vi "Set VI Allow Debugging Property.vi"() -> ()   [LabVIEW 2016]
doc: "A wrapper engine for setting separate compiled code for all VIs in a folder."
uses:
  <vilib>/Utility/error.llb/DialogType.ctl
  SLL Queued State Machine/Queue Driver/Create Queue.vi
  SLL Queued State Machine/Queue Driver/Enqueue an Item to Queue.vi
  SLL Queued State Machine/Queue Driver/Dequeue Queue.vi
  SLL Queued State Machine/Queue Driver/Enqueue N Items.vi
  SLL Queued State Machine/Queue Driver/Flush Queue.vi
  SLL Queued State Machine/Queue Driver/Release Queue.vi
  SLL Queued State Machine/SLL QSM.lvlib
panel:
  out "Progress":i32(slide) scale=0.0..10.0
  in  "Allow Debugging?":bool
  in  "Folder Path":path
  out "Status":string
  in  "Run":bool
  # "Set VI Allow Debugging Property"
  # "Sets the allow debugging property for the VIs in the folder"
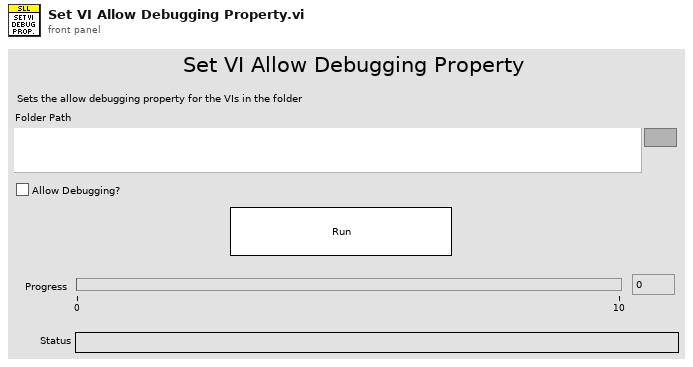
[diagram p1: front panel]
types:
  T1 = typedef "DialogType.ctl" = u16
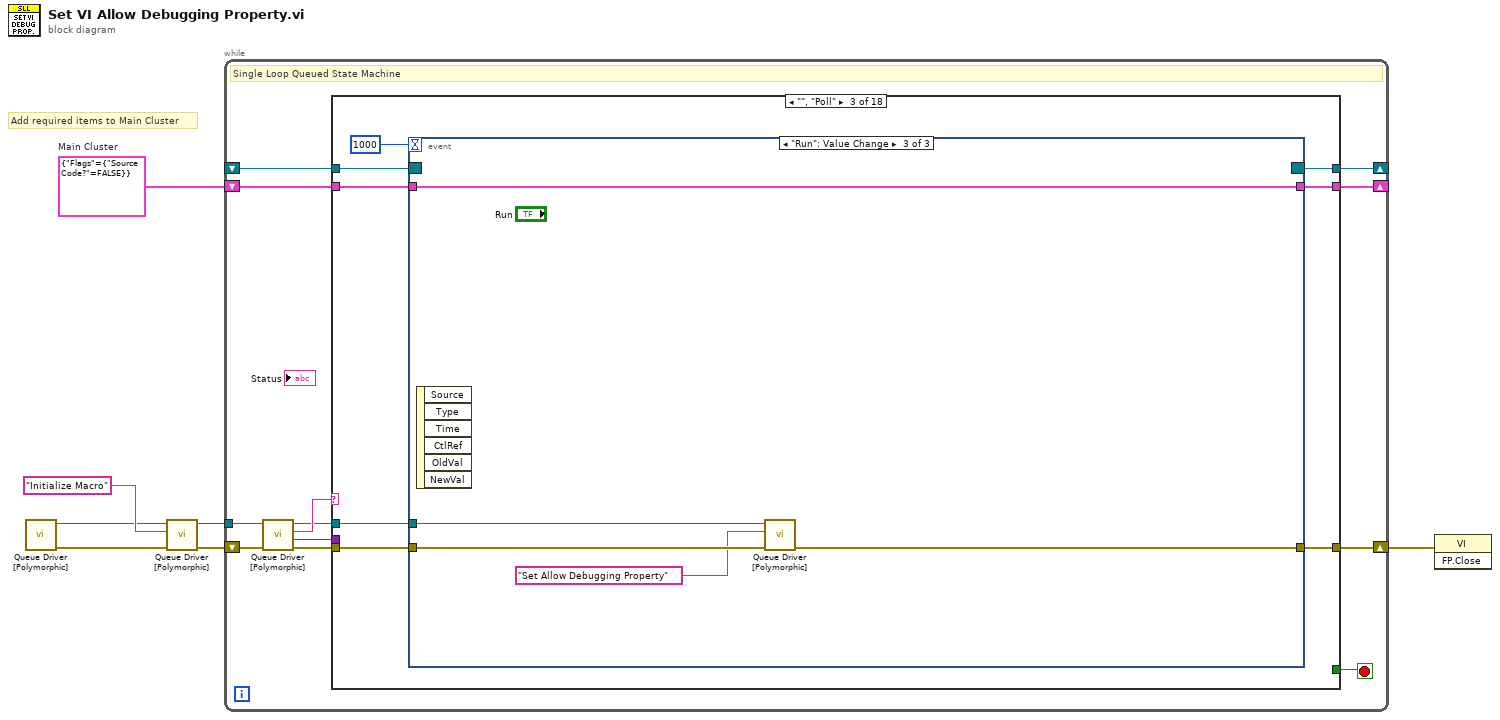
[diagram p0: block diagram]
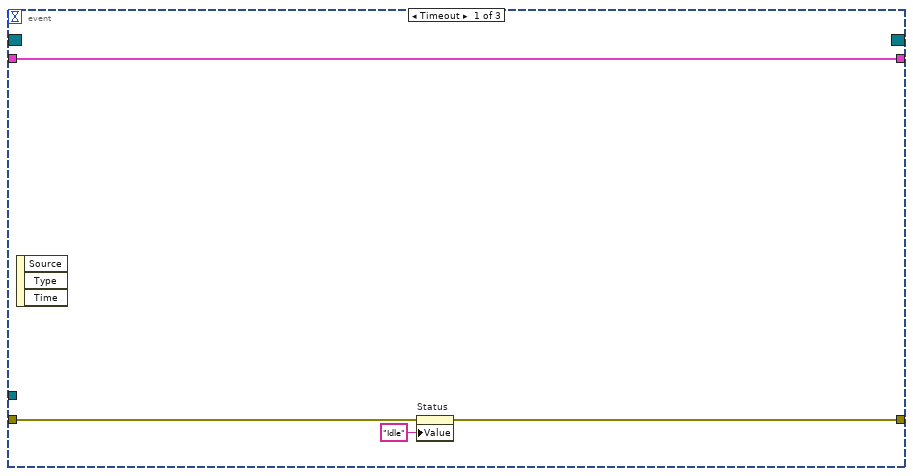
[diagram p4: hidden frame]
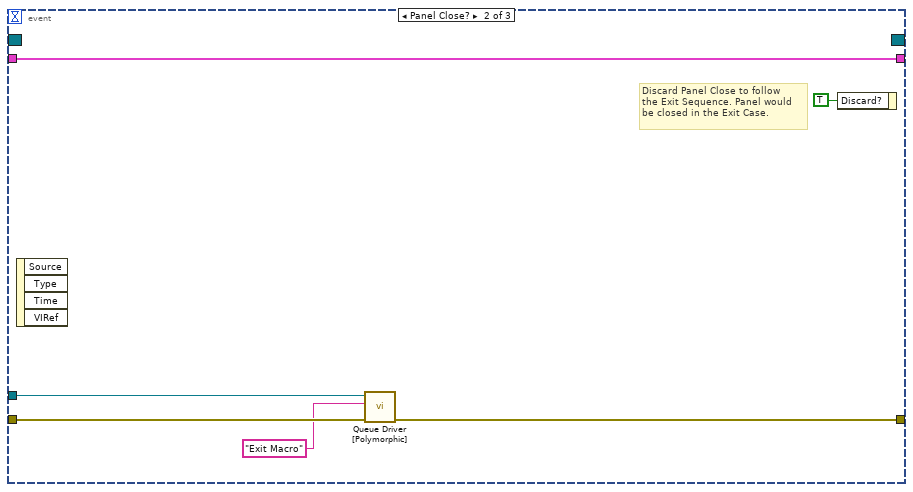
[diagram p5: hidden frame]
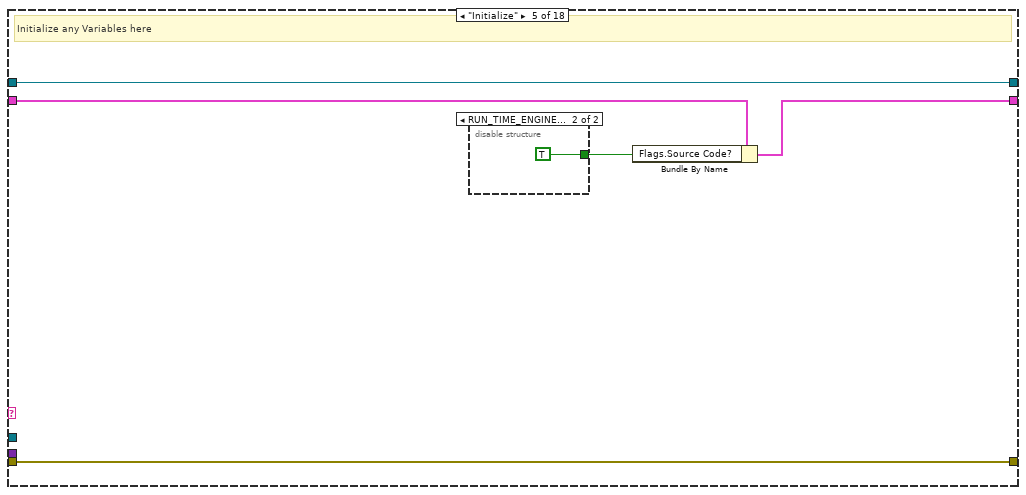
[diagram p7: hidden frame]
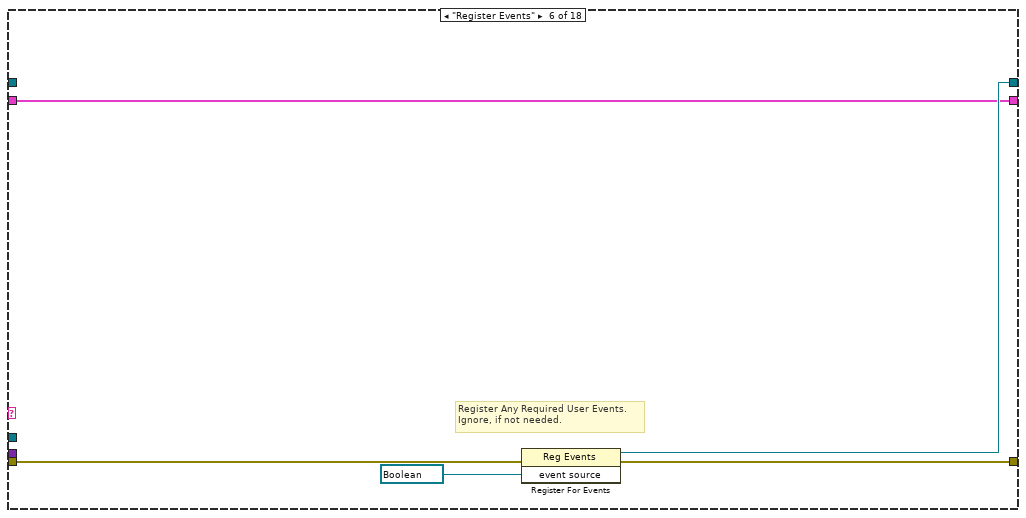
[diagram p9: hidden frame]
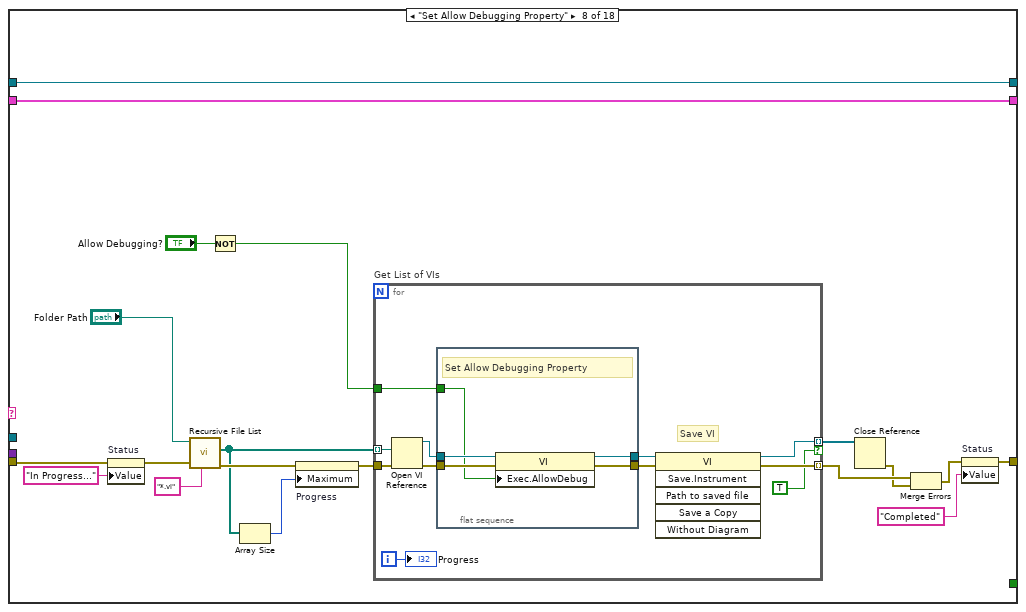
[diagram p11: hidden frame]
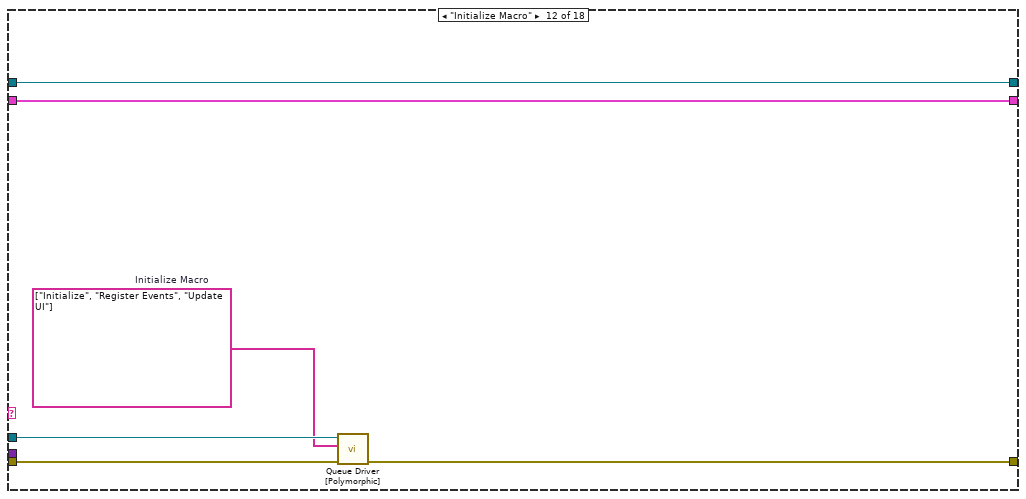
[diagram p15: hidden frame]
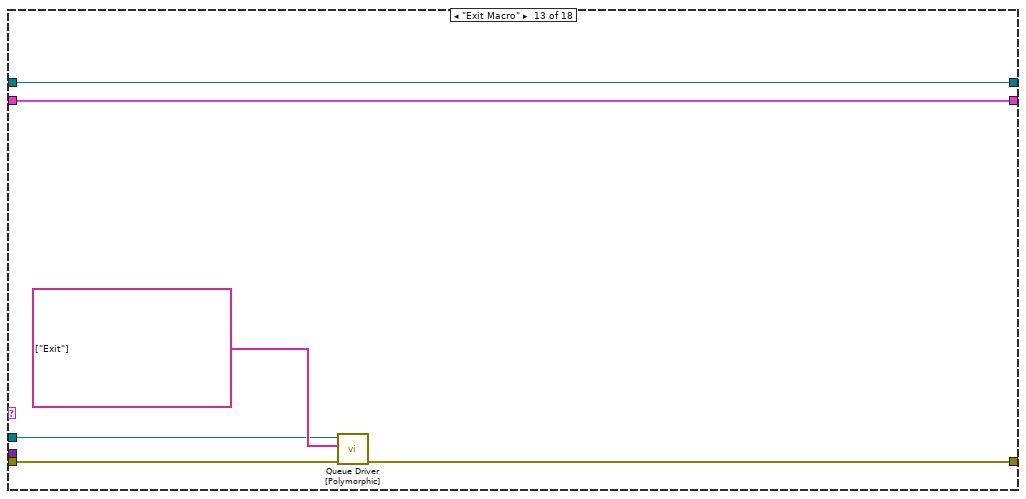
[diagram p16: hidden frame]
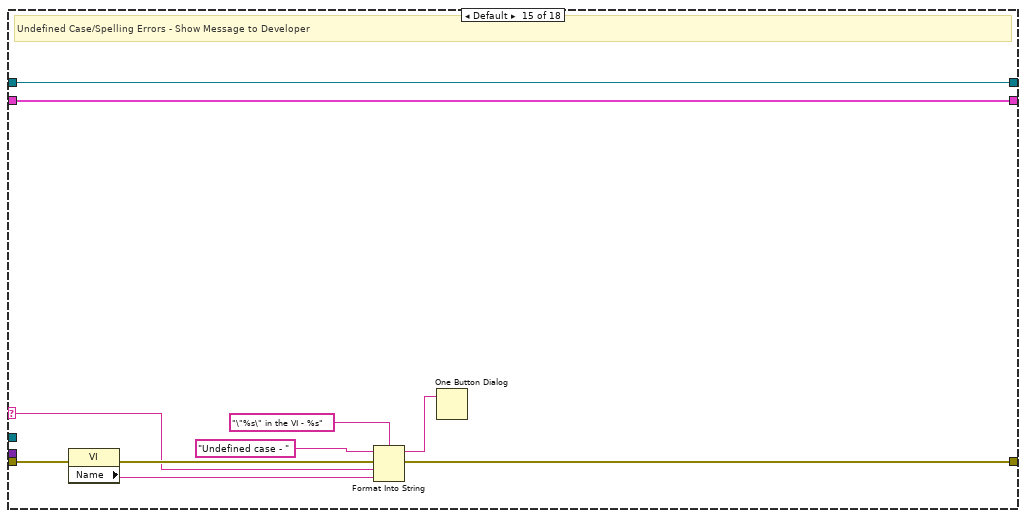
[diagram p18: hidden frame]
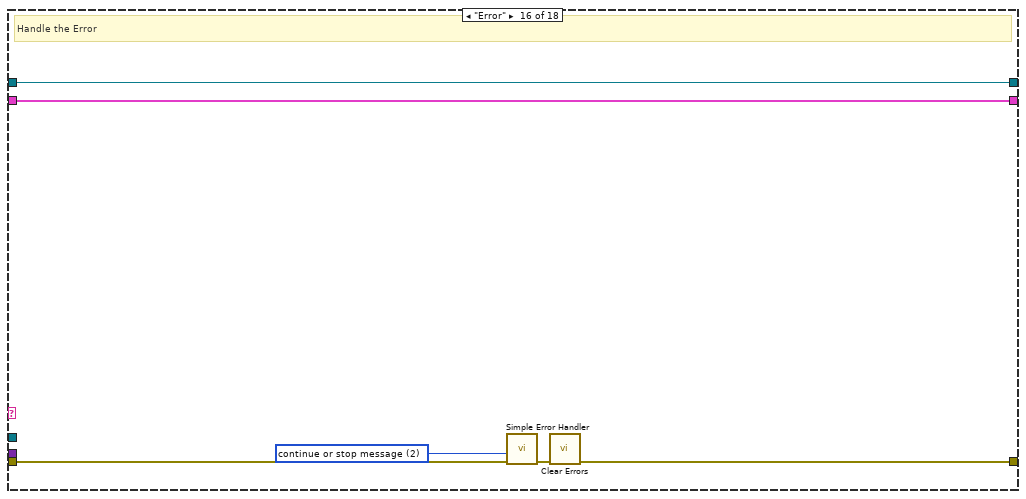
[diagram p19: hidden frame]
diagram:
  w5 = cluster{"Flags":cluster{"Source Code?":bool}} {"Flags"={"Source Code?"=FALSE}}  # Main Cluster
  # "Add required items to Main Cluster"
  n1 = call-poly "Queue Driver [Polymorphic].vi"() -> ("Error Out"=w7:errorcluster, "Queue Ref"=w3:refnum<queue>)  [unwired: 10 in]
  n2 = call-poly "Queue Driver [Polymorphic].vi"("Error In"=w7, "Item to Add"="Initialize Macro", "Queue Ref In"=w3) -> ("Error Out"=w6:errorcluster, "Queue Ref Out"=w2:refnum<queue>)  [unwired: 7 in]
  n3 = while "SLL Queued State Machine" {
    shift-right: [w17] -> w1
    shift-left: w6 -> [w19]
    shift-right: [w15] -> _
    shift-left: _ -> [w14]
    shift-right: [w13] -> _
    shift-left: w5 -> [w12]
    tunnel: w2 -> [w10]
    stop <- w16 stop-if-true
    # "Single Loop Queued State Machine"
    n4 = call-poly "Queue Driver [Polymorphic].vi"("Error In"=w19, "Queue Ref In"=w10) -> ("Error Out"=w18:errorcluster, "Data"=w8:variant, "Dequeue"=w11:string, "Queue Ref Out"=w9:refnum<queue>)  [unwired: 6 in]
    n5 = case "QSM Case Structure" shown="\"\", \"Poll\"" w11 {
      selector: w11 -> [_ _ _ _ _ _ _ _ _ _ _ _ _ _ w125 _ _ _]
      tunnel: w18 -> [w22 w25 w31 w51 w56 w62 w65 w79 w103 w106 w109 w113 w119 w124 w128 w140 w143 w156]
      tunnel: [w22 w25 w32 w51 w56 w61 w65 w81 w103 w106 w109 w112 w118 w124 w131 w138 w143 w152] -> w17
      tunnel: [_ _ _ _ _ _ _ _ _ _ _ _ _ _ _ _ _ TRUE] -> w16
      tunnel: [w21 w24 w30 w50 w55 w60 w64 w84 w102 w105 w108 w115 w121 w123 w134 w137 w142 w155] -> w15
      tunnel: w14 -> [w21 w24 w29 w50 w55 _ w64 w84 w102 w105 w108 w115 w121 w123 w134 w137 w142 w155]
      tunnel: [w20 w23 w27 w49 w52 w59 w63 w83 w101 w104 w107 w114 w120 w122 w133 w136 w141 w154] -> w13
      tunnel: w12 -> [w20 w23 w28 w49 w53 w59 w63 w83 w101 w104 w107 w114 w120 w122 w133 w136 w141 w154]
      tunnel: w9 -> [_ _ w26 _ _ _ _ _ _ _ _ w111 w116 _ _ _ _ w145]
      tunnel: w8 -> [_ _ _ _ _ _ _ _ _ _ _ _ _ _ _ _ _ _]
      frame "/--------------- Read Me -----------------/" {
        # "General Purpose Queue Based State Machine for Any Use Case (main application, module, pop up message etc)\n\nAdvantages:\n1. No Need to Pass Queue References between Queue Driver VIs.\n2. This template can be safely used in multiple parallel running modules without any issues.\n3. This template can also be safely used even in cases where the VI is configured to be a Clone, where multiple \ninstances of the VI could be executing concurrently.\n\nHow to Use:\n1. Add necessary items to the Main Cluster.\n2. Use the Polymorphic Queue Driver for doing any queue operations. There is no need to pass the queue driver\nreference, as the Queue Driver automatically infers the reference based on the VI instance from which it is called.\n3. Add any required user events in the \"Register Events\" case. Ignore if not needed.\n4. Use \"Sequences\" section for defining any list of state calls, which could be used in multiple places. \nEg: Initialize Sequence, might be needed if we need to any reinitialization."
      }
      frame "/------------------ Poll -------------------/" {
      }
      frame "", "Poll" {
        n6 = event shown="[2] \"Run\": Value Change" {
          selector: w29 -> [_ _ _]
          dyn-events: [_ _ _] -> w30
          timeout: 1000 -> [_ _ _]
          tunnel: [w34 w42 w47] -> w32
          tunnel: w31 -> [w35 w43 w48]
          tunnel: w28 -> [w37 w41 w46]
          tunnel: [w37 w41 w46] -> w27
          tunnel: w26 -> [_ w38 w45]
          event Timeout {
            n7 = event-data() -> ()  [unwired: 1 in, 3 out]
            n8 = property on="Status" class="Str"(error in=w35, "Value"="Idle" ("Status")) -> (error out=w34:errorcluster)  [unwired: 1 in, 1 out]
          }
          event Panel Close? {
            # "Discard Panel Close to follow\nthe Exit Sequence. Panel would\nbe closed in the Exit Case."
            n9 = event-data() -> ()  [unwired: 1 in, 4 out]
            n10 = call-poly "Queue Driver [Polymorphic].vi"("Error In"=w43, "Item to Add"="Exit Macro" ("Enqueue"), "Queue Ref In"=w38) -> ("Error Out"=w42:errorcluster)  [unwired: 7 in, 1 out]
            n11 = event-data("Discard?"=TRUE) -> ()  [unwired: 1 in, 1 out]
          }
          event "Run": Value Change {
            n12 = event-data() -> ()  [unwired: 1 in, 6 out]
            n13 = call-poly "Queue Driver [Polymorphic].vi"("Error In"=w48, "Item to Add"="Set Allow Debugging Property", "Queue Ref In"=w45) -> ("Error Out"=w47:errorcluster)  [unwired: 7 in, 1 out]
          }
        }
      }
      frame "/--------------- Initialize -----------------/" {
      }
      frame "Initialize" {
        # "Initialize any Variables here"
        n14 = disable-structure shown="RUN_TIME_ENGINE==False" {
          disable-tunnel: [_ TRUE] -> w54
          frame condition #0 {
          }
          frame condition #1 (active) {
          }
        }
        n15 = Bundle By Name(cluster=w53, "Flags.Source Code?"=w54) -> (w52:cluster{"Flags":cluster{"Source Code?":bool}})
      }
      frame "Register Events" {
        # "Register Any Required User Events. \nIgnore, if not needed."
        n16 = register-events(error in=w62, refnum<vi> refnum ("event source")) -> (reference out=w60:refnum<event-registration>, error out=w61:errorcluster)  [unwired: 1 in]
      }
      frame "/---------- Custom Case Splitter ----------/" {
      }
      frame "Set Allow Debugging Property" {
        n17 = property on="Status" class="Str"(error in=w79, "Value"="In Progress..." ("Status")) -> (error out=w73:errorcluster)  [unwired: 1 in, 1 out]
        n18 = call <vilib>:"Recursive File List.vi"("pattern"="*.vi", "error in (no error)"=w73, "Folder Path"="Folder Path") -> ("error out"=w69:errorcluster, "All Files in Dir"=w67:path[])  [unwired: 4 in, 3 out]
        n19 = Not(x="Allow Debugging?") -> (.not. x?=w74:bool)
        n20 = Array Size(array=w67) -> (size(s)=w66:i32)
        n21 = property on="Progress" class="Slide (strict)"(error in=w69, "Maximum"=w66) -> (error out=w68:errorcluster)  [unwired: 1 in, 1 out]
        n22 = for "Get List of VIs" {
          tunnel: [w94] -> w78 mode=indexing if=TRUE
          tunnel: w67 -> [w91] mode=indexing
          tunnel: w68 -> [w93]
          tunnel: [w95] -> w76 mode=indexing
          tunnel: w74 -> [w90]
          i -> [w85]
          # "Save VI"
          n23 = Open VI Reference(vi path=w91, error in (no error)=w93) -> (vi reference=w89:refnum<vi>, error out=w88:errorcluster)  [unwired: 4 in]
          n24 = flat-sequence {
            tunnel: w89 -> [w98]
            tunnel: w88 -> [w100]
            tunnel: [w99] -> w87
            tunnel: [w97] -> w86
            tunnel: w90 -> [w96]
            frame #0 {
              # "Set Allow Debugging Property"
              n25 = property class="VI"(reference=w98, error in=w100, "Exec.AllowDebug"=w96) -> (reference out=w97:refnum<vi>, error out=w99:errorcluster)
            }
          }
          n26 = invoke class="VI" method="Save.Instrument"(reference=w86, error in=w87) -> (reference out=w94:refnum<vi>, error out=w95:errorcluster)  [unwired: 4 in, 4 out]
          "Progress" <- w85
        }
        n27 = Close Reference(reference=w78) -> (error out=w75:errorcluster)  [unwired: 1 in]
        n28 = Merge Errors(w76, w75) -> (w70:errorcluster)
        n29 = property on="Status" class="Str"(error in=w70, "Value"="Completed" ("Status")) -> (error out=w81:errorcluster)  [unwired: 1 in, 1 out]
      }
      frame "/-------------- User Interface --------------/" {
        # "Duplicate this case to create additional case splitters for readability"
      }
      frame "Update UI" {
        # "Update Front Panel Controls in this Case"
      }
      frame "/----------------- Macros -----------------/" {
      }
      frame "Initialize Macro" {
        w110 = string[] ["Initialize", "Register Events", "Update UI"]  # Initialize Macro
        n30 = call-poly "Queue Driver [Polymorphic].vi"("Error In"=w113, "Enqueue N"=w110, "Queue Ref In"=w111) -> ("Error Out"=w112:errorcluster)  [unwired: 7 in, 1 out]
      }
      frame "Exit Macro" {
        n31 = call-poly "Queue Driver [Polymorphic].vi"("Error In"=w119, "Enqueue N"=string[] ["Exit"], "Queue Ref In"=w116) -> ("Error Out"=w118:errorcluster)  [unwired: 7 in, 1 out]
      }
      frame "/-------------- Error Handler--------------/" {
      }
      frame Default {
        # "Undefined Case/Spelling Errors - Show Message to Developer"
        n32 = property class="VI"(error in=w128) -> (error out=w127:errorcluster, "Name"=w126:string)  [unwired: 1 in, 1 out]
        n33 = Format Into String(format string="\"%s\" in the VI - %s" ("message"), initial string="Undefined case - ", error in=w127, w125, w126) -> (resulting string=w129:string, error out=w131:errorcluster)
        n34 = One Button Dialog(message=w129) -> ()  [unwired: 1 in, 1 out]
      }
      frame "Error" {
        w135 = T1 2 items=["no dialog", "OK message", "continue or stop message", "OK message + warnings", "continue/stop + warnings"] ("type of dialog (OK msg:1)")
        # "Handle the Error"
        n35 = call <vilib>:"Simple Error Handler.vi"("type of dialog (OK msg:1)"=w135, "error in (no error)"=w140) -> ("error out"=w139:errorcluster)  [unwired: 3 in, 4 out]
        n36 = call <vilib>:"Clear Errors.vi"("error in (no error)"=w139) -> ("error out"=w138:errorcluster)  [unwired: 5 in, 1 out]
      }
      frame "/------------------- Exit --------------------/" {
      }
      frame "Exit" {
        n37 = call-poly "Queue Driver [Polymorphic].vi"("Error In"=w156, "Queue Ref In"=w145) -> ("Error Out"=w157:errorcluster, "Queue Ref Out"=w144:refnum<queue>)  [unwired: 7 in, 1 out]
        n38 = Unbundle By Name(w154) -> ("Flags.Source Code?"=w147:bool)
        n39 = call-poly "Queue Driver [Polymorphic].vi"("Error In"=w157, "Queue Ref In"=w144) -> ("Error Out"=w153:errorcluster)  [unwired: 9 in]
        n40 = Call Chain() -> (call chain=w151:string[])
        n41 = Array Size(array=w151) -> (size(s)=w150:i32)
        n42 = Equal?(x=w150, y=1) -> (x = y?=w148:bool)
        n43 = And(x=w147, y=w148) -> (x .and. y?=w146:bool)
        n44 = case "Skip Panel Close when in Source\nCode and is the top most caller" shown="True" w146 {
          tunnel: w153 -> [w160 w162]
          tunnel: [w161 w162] -> w152
          frame False {
            # "Close Panel"
            n45 = invoke class="VI" method="FP.Close"() -> (error out=w159:errorcluster)  [unwired: 3 in, 2 out]
            n46 = Merge Errors(w160, w159) -> (w161:errorcluster)
          }
          frame True {
            # "Do Not Close Panel"
          }
        }
      }
    }
  }
  n47 = invoke class="VI" method="FP.Close"(error in=w1) -> ()  [unwired: 2 in, 3 out]
